vi "副屏设置全局变量.vi"() -> ()   [LabVIEW 2016, in "副屏.lvlib"]
panel:
  in  "藻密度":bool=TRUE caption="氨氮禁用"
  in  "叶绿素a":bool=TRUE caption="氨氮禁用"
  in  "启用副屏":bool caption="氨氮禁用"
  in  "底部状态栏显示信息":string="一体化微型水质监测系统"
  in  "流速":bool caption="氨氮禁用"
  in  "瞬时流量":bool caption="氨氮禁用"
  in  "湿度":bool=TRUE caption="氨氮禁用"
  in  "水位":bool caption="氨氮禁用"
  in  "室温":bool=TRUE caption="氨氮禁用"
  in  "CODCr":bool caption="氨氮禁用"
  in  "CODMn":bool caption="氨氮禁用"
  in  "总氮":bool caption="氨氮禁用"
  in  "总磷":bool caption="氨氮禁用"
  in  "氨氮":bool caption="氨氮禁用"
  in  "Turb":bool caption="氨氮禁用"
  in  "Cond":bool caption="氨氮禁用"
  in  "DO":bool caption="氨氮禁用"
  in  "pH":bool caption="氨氮禁用"
  in  "水温":bool caption="氨氮禁用"
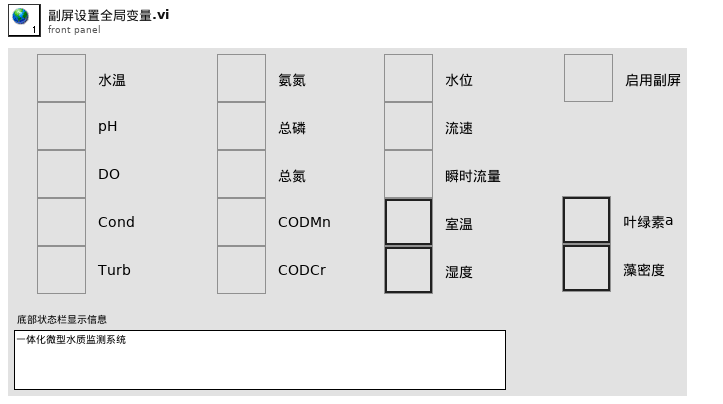
[diagram p1: front panel]
diagram:
